vi "MakeBar-File.vi"(2 "position offset":i32, 3 "path":path) -> (0 "output array":u8[](array[numeric]), 1 "offset":i32)   [LabVIEW 2018]
uses:
  <vilib>/express/express analysis/Spectral/Block/exnSpectralBlock spectral measurements RMS poly.vi
  <vilib>/express/express analysis/Spectral/Block/exnSpectralBlock spectral measurements RMS DDT.vi
  <vilib>/express/express analysis/Spectral/XNode/ExpressSpectralMeasurementsBlockNode.xnode
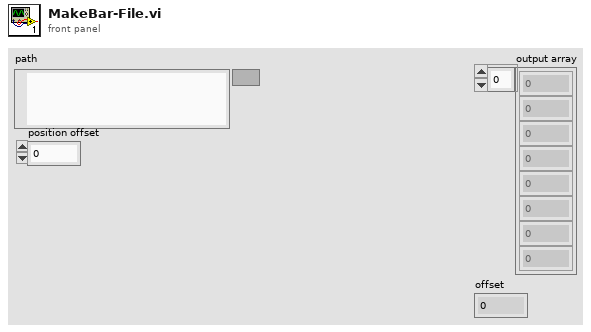
[diagram p1: front panel]
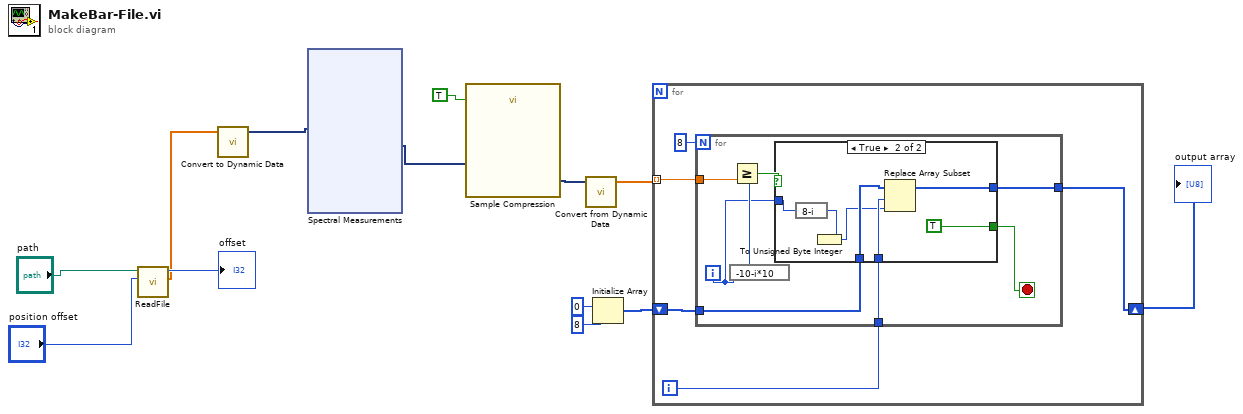
[diagram p0: block diagram]
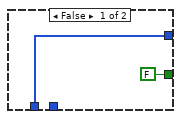
[diagram p2: hidden frame]
diagram:
  n1 = call "ReadFile.vi"("position offset"="position offset", "path"="path") -> ("Y"=w1:dbl[], "offset"=→"offset":i32)  [unwired: 8 in]
  n2 = call "Convert to Dynamic Data"("Array"=w1) -> ("Dynamic Data Type"=w3:dynamicdata)  [unwired: 3 in]
  n3 = xnode "Spectral Measurements"("Signals"=w3) -> ("FFT - (RMS)"=w8:dynamicdata)  [unwired: 1 in, 2 out]
  n4 = call "Sample Compression"("Enable"=TRUE, "Signals"=w8) -> ("Maximum"=w7:dynamicdata)  [unwired: 7 in, 2 out]
  n5 = call "Convert from Dynamic Data"("Dynamic Data Type"=w7) -> ("Array"=w6:dbl[])  [unwired: 3 in]
  n6 = Initialize Array(u8 0 ("element"), 8 ("dimension size")) -> (w10:u8[])
  n7 = for {
    tunnel: w6 -> [w17] mode=indexing
    shift-right: [w14] -> w9
    shift-left: w10 -> [w15]
    i -> [w16]
    n8 = for {
      N: 8 -> [_]
      tunnel: w17 -> [w25]
      tunnel: w16 -> [w23]
      tunnel: w15 -> [w21]
      tunnel: [w22] -> w14
      i -> [w24]
      stop <- w19 stop-if-true
      n9 = expression code="-10-i*10"(w24) -> (w26:i32)
      n10 = Greater Or Equal?(x=w25, y=w26) -> (x >= y?=w20:bool)
      n11 = case shown="True" w20 {
        tunnel: w24 -> [_ w34]
        tunnel: w23 -> [_ w35]
        tunnel: w21 -> [w28 w33]
        tunnel: [w28 w30] -> w22
        tunnel: [FALSE TRUE] -> w19
        frame False {
        }
        frame True {
          n12 = expression code="8-i"(w34) -> (w32:i32)
          n13 = To Unsigned Byte Integer(number=w32) -> (unsigned 8bit integer=w31:u8)
          n14 = Replace Array Subset(array=w33, new element=w31, index=w35) -> (w30:u8[])
        }
      }
    }
  }
  "output array" <- w9
